vi "Plugin-001-MaterialTest.vi"(0 "Configuration Page":refnum<class "Material-ConfigPage.lvclass">, 11 "error in":errorcluster) -> (15 "error out":errorcluster)   [LabVIEW 2013, in "Material-RunTest.lvclass"]
doc: "DisplayName=\"Deploy Configuration Template\"\nDescription=\"This VI serves as a template page for the Deploy Configuration UI.\""
uses:
  Plugins/Run Material Test/Material-RunTest.lvclass
  Material-ConfigPage.lvclass
  Reuse Library/featherweight/Core/Sequencer/FTW-Sequencer.lvclass/FTW-Sequencer.ctl
  Plugins/Run Material Test/Material-RunTest.lvclass/Material-RunTest.ctl
  <vilib>/Utility/miscctls.llb/LVPointTypeDef.ctl
  Reuse Library/featherweight/Core/Regex/FTW-Regex.vi
  Reuse Library/featherweight/Core/Error/FTW-ERR-StatusException.vi
  Reuse Library/featherweight/Core/Error/FTW-ERR-ThrowError.vi
  Reuse Library/featherweight/Core/Sequencer/FTW-Sequencer.lvclass
  Reuse Library/featherweight/Core/Messaging/Message.Actor/FTW-Message-Actor.lvclass
  <instrlib>/Keyence LK-G5000/Keyence LK-G5000.lvlib
  <instrlib>/Keyence LK-G5000/Public/Constant/Comm Interface.ctl
  Plugins/Motion Control/Motion-ControlAll.lvclass
  Reuse Library/Database API/Database-API.lvclass
panel:
  out "Overall Sheet Passed?":bool
  out "Total Average Thickness of Sheet":dbl format="%_6g"
  out "Average Thickness Line 3":dbl format="%_5g"
  out "Average Thickness Line 2":dbl format="%_5g"
  out "Average Thickness Line 1":dbl format="%_5g"
  out "Thickness Measured Real Time":sgl format="%_6g"
  in  "Begin Test":bool
  out "Line 3 test passed?":bool
  out "Line 2 test passed?":bool
  out "Line 1 test passed?":bool
  out "Mixed Signal Graph":T1(graph)
  out "Message Received":string
  # "Inputs"
  # "Outputs"
  # "First Plugin"
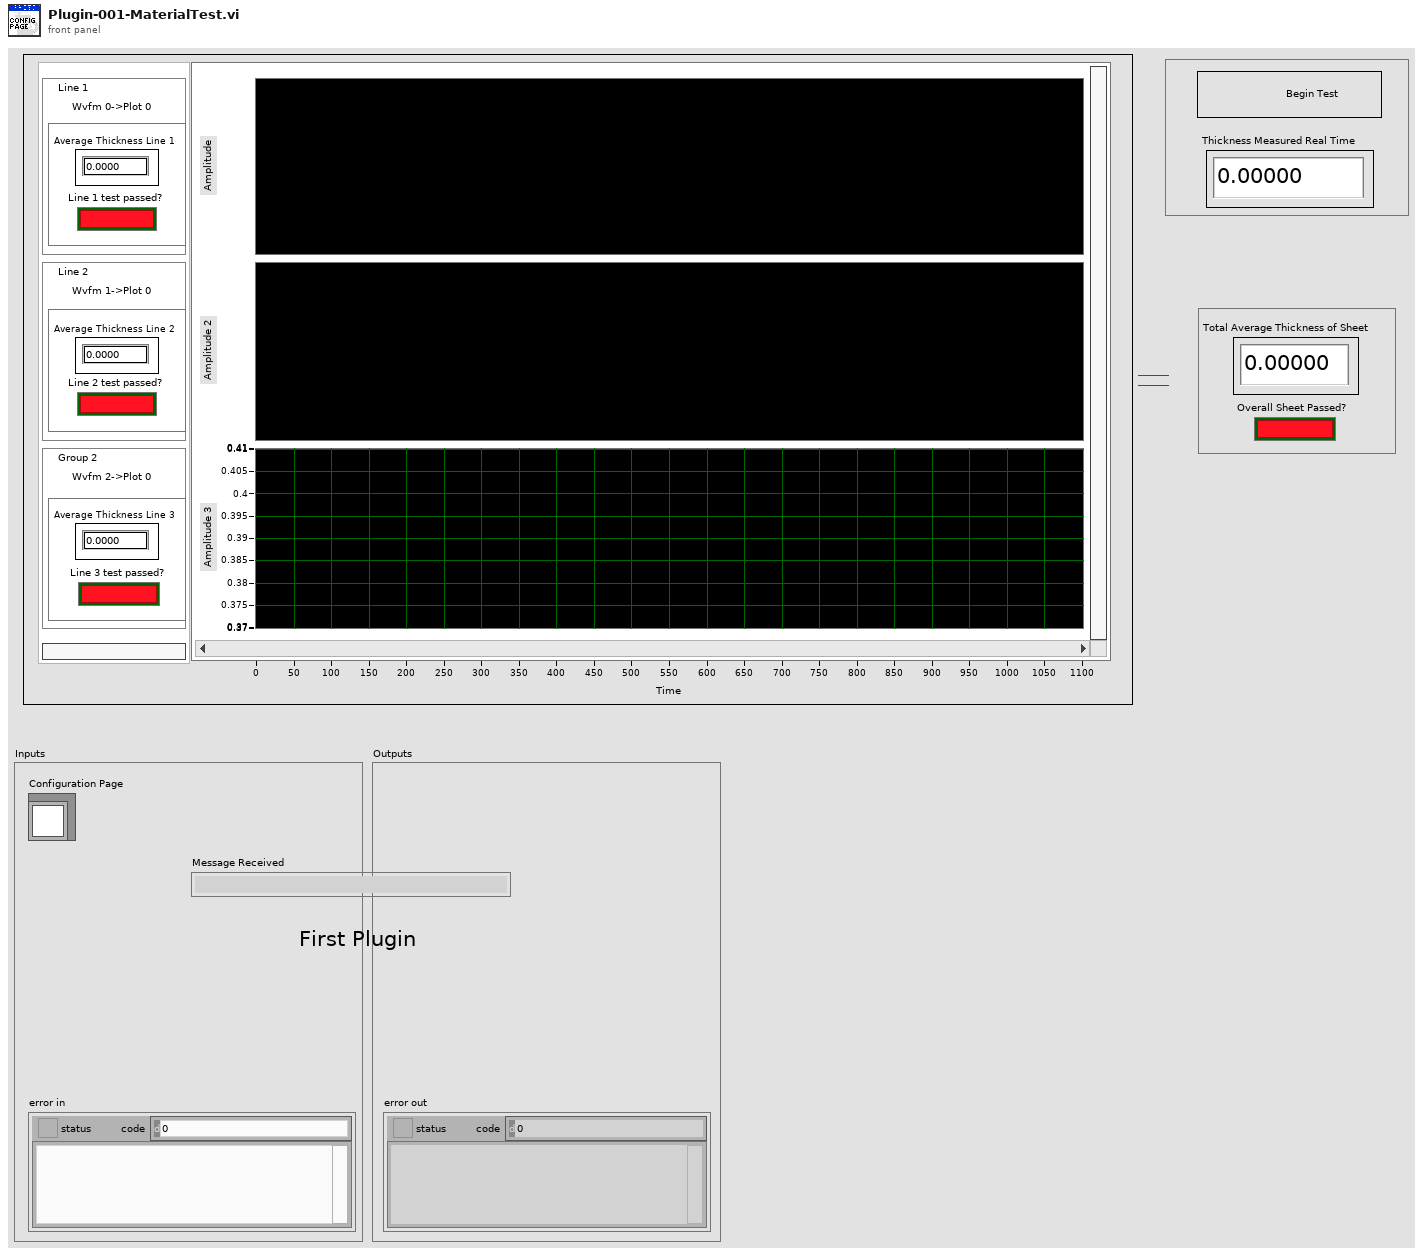
[diagram p1: front panel]
types:
  T1 = cluster{waveform(sgl), waveform(sgl), waveform(sgl)}
  T2 = typedef "Keyence LK-G5000.lvlib/Comm Interface.ctl" = enum8{"USB", "ETHERNET"}
  T3 = typedef "LVPointTypeDef.ctl" = cluster{"Horizontal":i16, "Vertical":i16}
  T4 = cluster{"PageCommands":refnum<event-registration>}
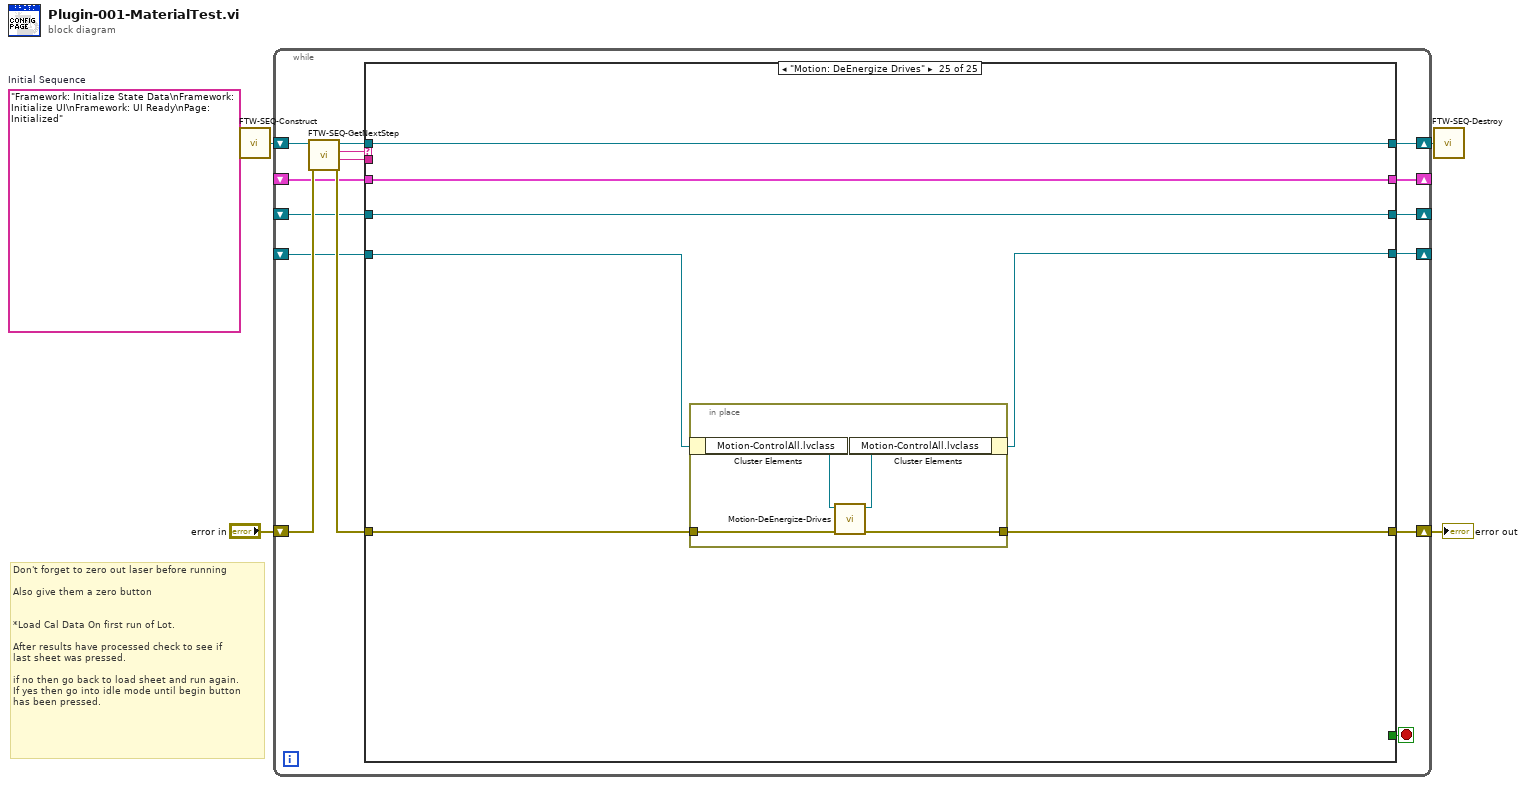
[diagram p0: block diagram]
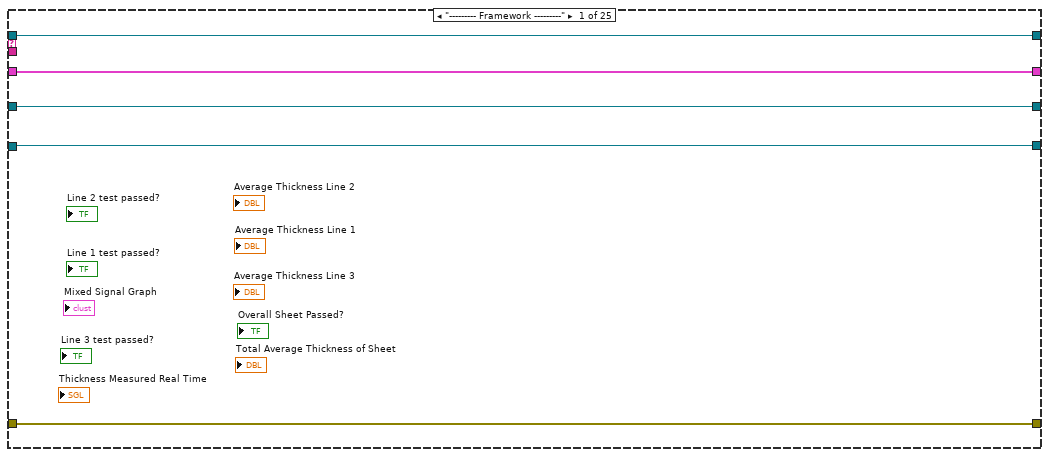
[diagram p2: hidden frame]
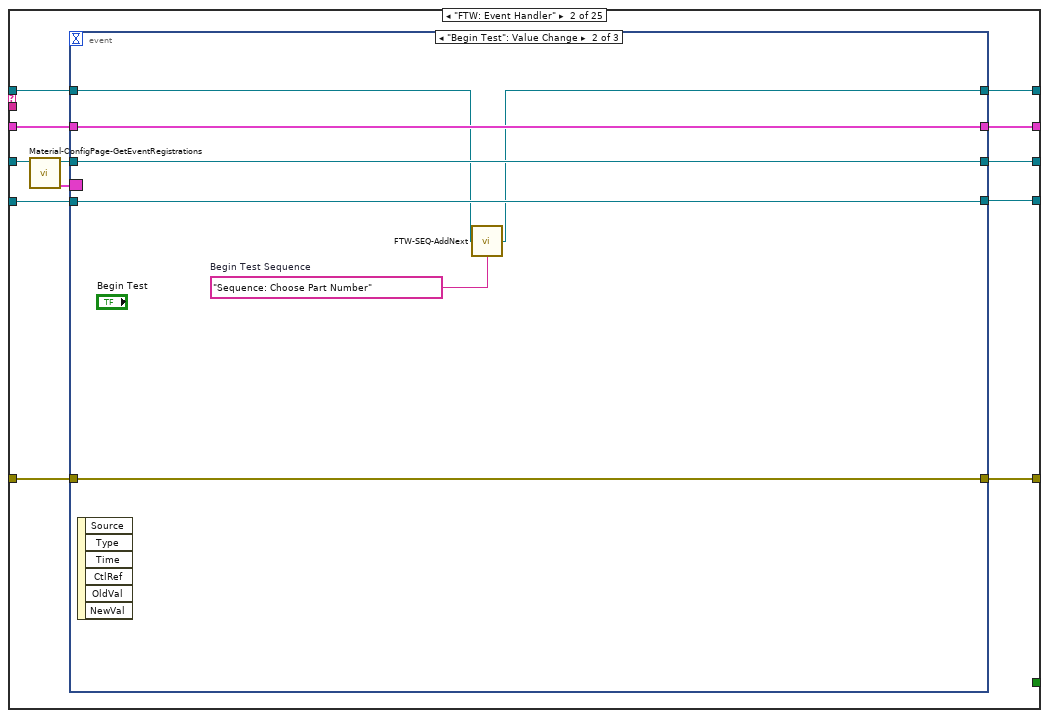
[diagram p3: hidden frame]
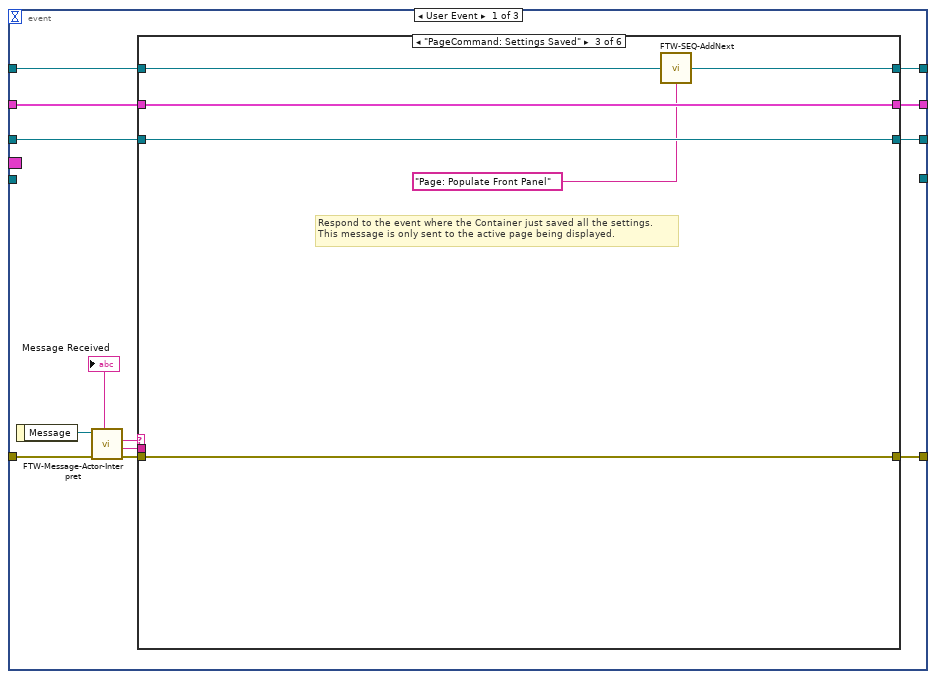
[diagram p4: hidden frame]
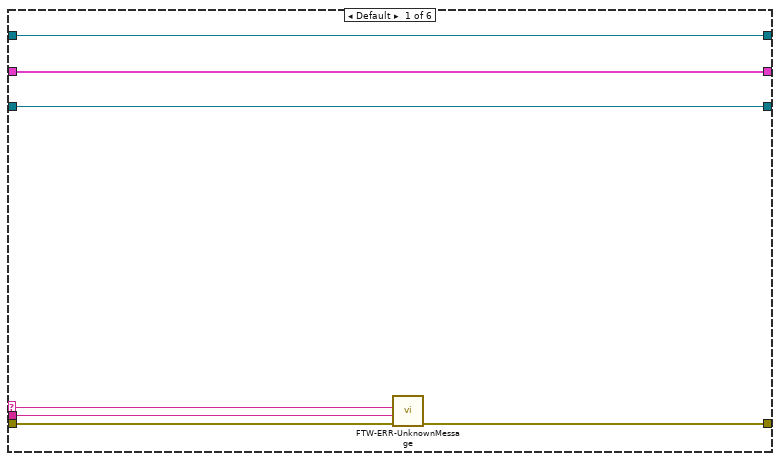
[diagram p5: hidden frame]
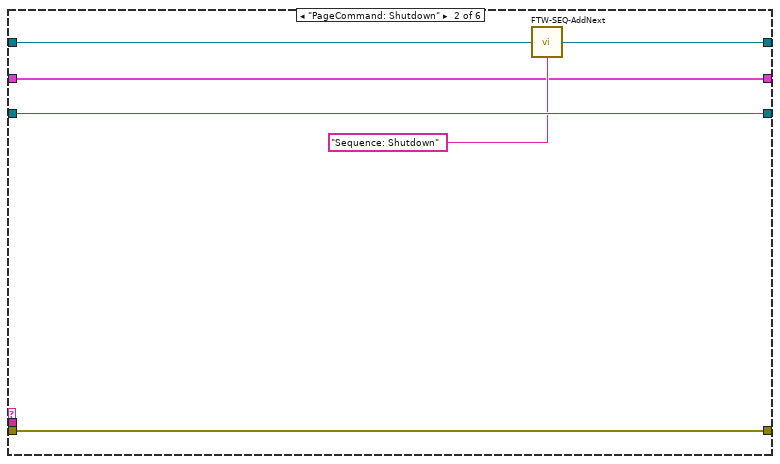
[diagram p6: hidden frame]
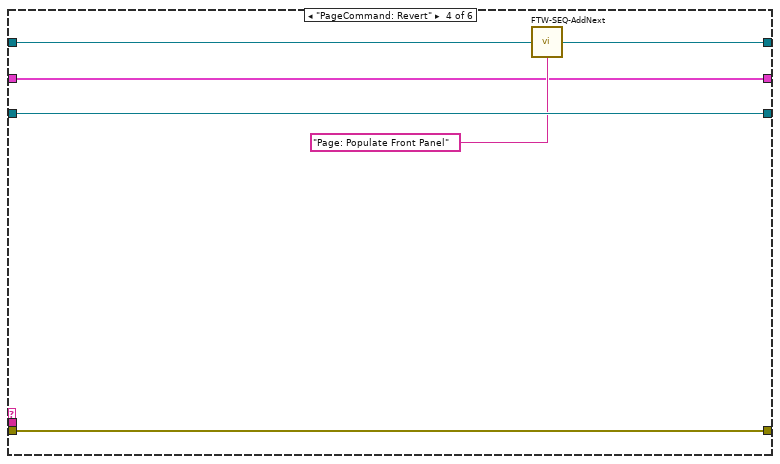
[diagram p7: hidden frame]
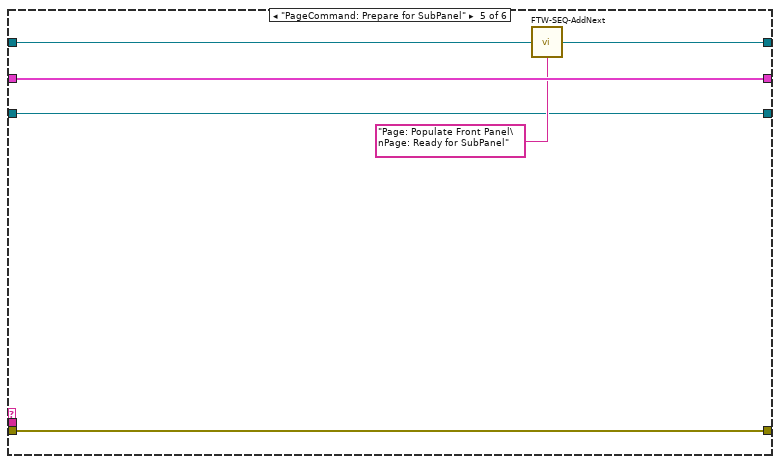
[diagram p8: hidden frame]
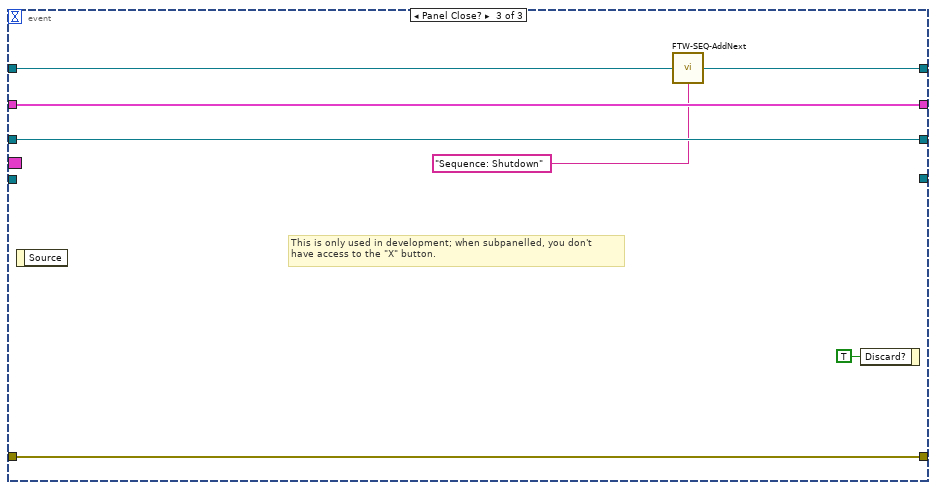
[diagram p10: hidden frame]
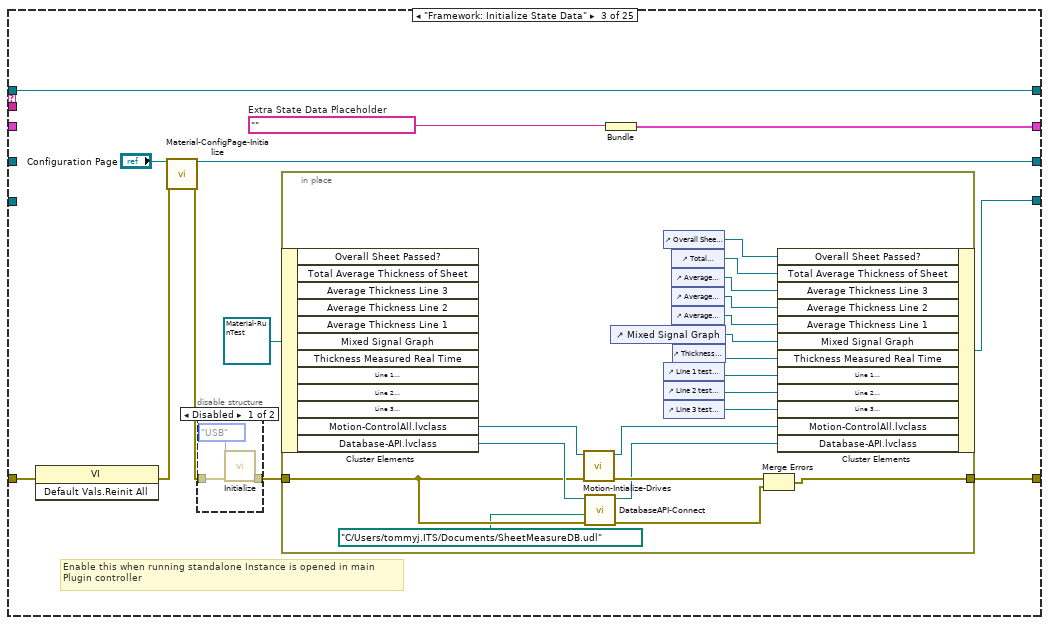
[diagram p11: hidden frame]
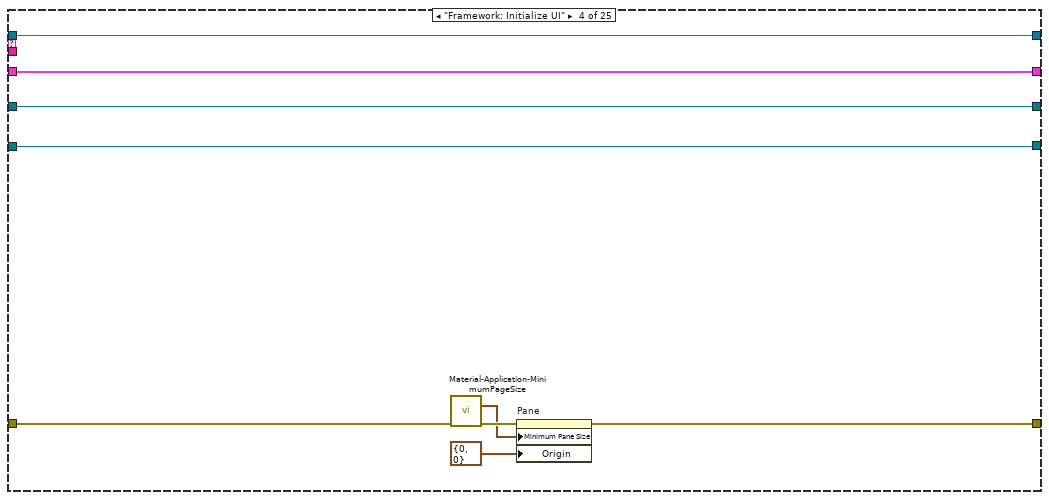
[diagram p13: hidden frame]
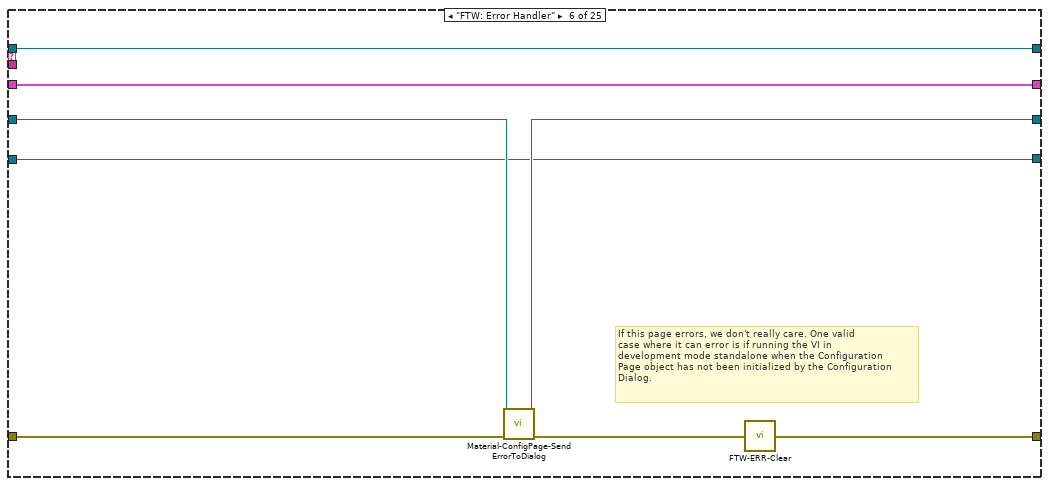
[diagram p15: hidden frame]
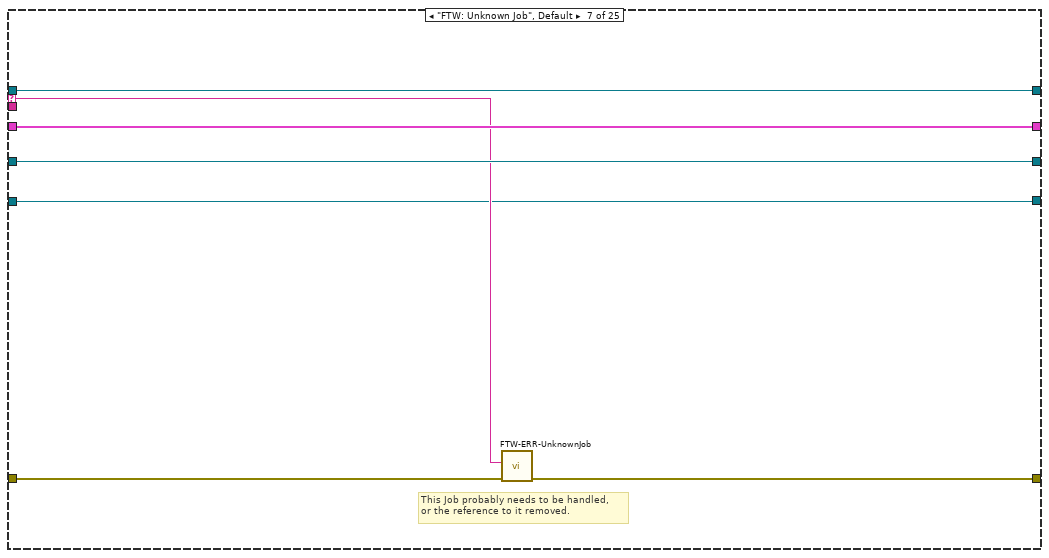
[diagram p16: hidden frame]
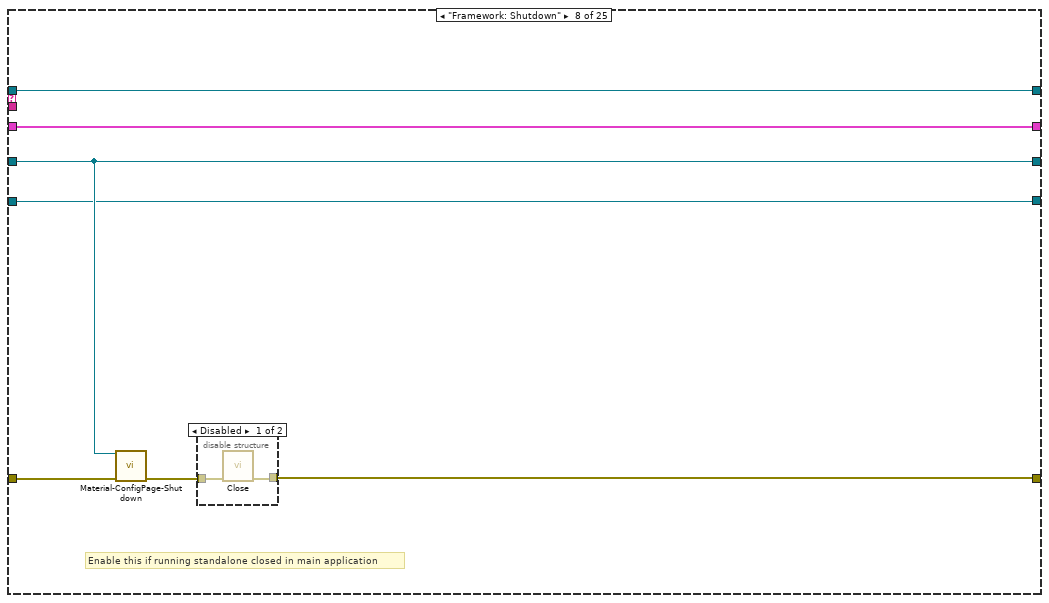
[diagram p17: hidden frame]
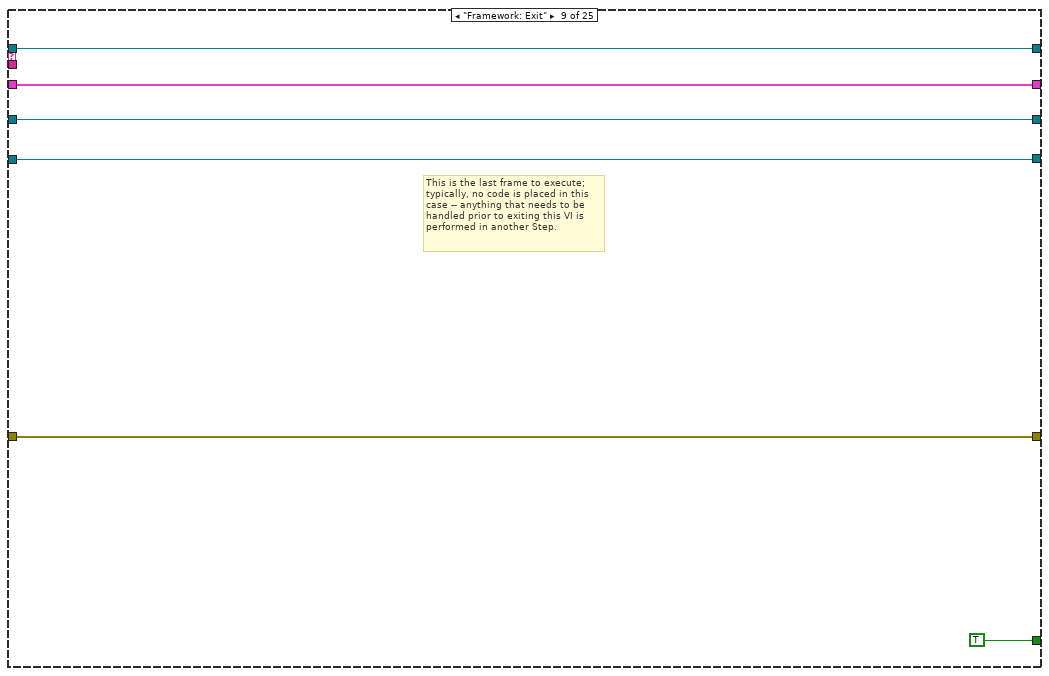
[diagram p19: hidden frame]
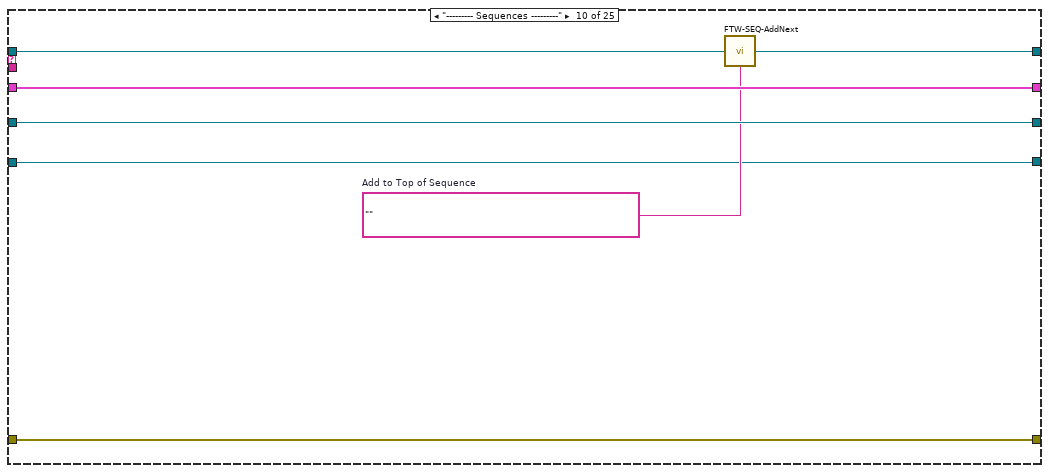
[diagram p20: hidden frame]
diagram:
  w5 = "Framework: Initialize State Data\nFramework: Initialize UI\nFramework: UI Ready\nPage: Initialized"  # Initial Sequence
  # "Don't forget to zero out laser before running\n\nAlso give them a zero button\n\n\n*Load Cal Data On first run of Lot.\n\nAfter results have processed check to see if\nlast sheet was pressed. \n\nif no then go back to load sheet and run again. \nIf yes then go into idle mode until begin button\nhas been pressed."
  n1 = call "FTW-SEQ-Construct.vi"("Initial Sequence"=w5) -> ("Sequencer"=w4:refnum<class "FTW-Sequencer.lvclass">)
  n2 = while {
    shift-right: [w18] -> w3
    shift-left: w4 -> [w9]
    shift-right: [w19] -> w2
    shift-left: "error in" -> [w17]
    shift-right: [w13] -> _
    shift-left: _ -> [w12]
    shift-right: [w11] -> _
    shift-left: _ -> [w10]
    shift-right: [w7] -> _
    shift-left: _ -> [w6]
    stop <- w14 stop-if-true
    n3 = call "FTW-SEQ-GetNextStep.vi"("error in"=w17, "Sequencer"=w9) -> ("error out"=w20:errorcluster, "Job Data"=w8:string, "Current Job"=w15:string, "Sequencer out"=w16:refnum<class "FTW-Sequencer.lvclass">)  [unwired: 6 in]
    n4 = case shown="\"Motion: DeEnergize Drives\"" w15 {
      selector: w15 -> [_ _ _ _ _ _ w157 _ _ _ _ _ _ _ _ _ _ _ _ _ _ _ _ _ _]
      tunnel: [w23 w35 w101 w138 w147 w154 w159 w163 w176 w184 w191 w197 w209 w230 w251 w258 w265 w276 w289 w295 w299 w308 w310 w315 w326] -> w19
      tunnel: w20 -> [w23 w34 w106 w139 w147 w151 w160 w167 w176 w184 w191 w200 w208 w233 w253 w260 w267 w278 w289 w296 w299 w309 w310 w318 w329]
      tunnel: w16 -> [w24 w37 w109 w137 w144 w149 w162 w168 w174 w181 w188 w202 w214 w235 w254 w261 w268 w273 w286 w292 w302 w304 w313 w320 w331]
      tunnel: [w24 w36 w109 w137 w144 w149 w162 w168 w174 w180 w187 w201 w214 w235 w254 w261 w268 w274 w286 w292 w302 w304 w313 w320 w331] -> w18
      tunnel: [_ _ _ _ _ _ _ _ TRUE _ _ _ _ _ _ _ _ _ _ _ _ _ _ _ _] -> w14
      tunnel: [w25 w33 w110 w142 w146 w155 w161 w169 w177 w185 w192 w204 w216 w237 w256 w263 w270 w280 w288 w297 w301 w307 w314 w321 w332] -> w13
      tunnel: w12 -> [w25 w31 _ w142 w146 w155 w161 w169 w177 w185 w192 w204 w216 w237 w256 w263 w270 w280 w288 w297 w301 w307 w314 w321 w332]
      tunnel: [w22 w32 w102 w135 w145 w152 w158 w166 w175 w183 w190 w203 w215 w236 w255 w262 w269 w279 w287 w293 w300 w305 w312 w319 w330] -> w11
      tunnel: w10 -> [w22 w30 _ w135 w145 w153 w158 w166 w175 w183 w190 w203 w215 w236 w255 w262 w269 w279 w287 w294 w300 w306 w312 w319 w330]
      tunnel: w8 -> [_ _ _ _ _ _ _ _ _ _ _ _ _ _ _ _ _ _ _ _ _ _ _ _ _]
      tunnel: [w21 w26 w99 w134 w143 w148 w156 w165 w173 w179 w186 w198 w210 w229 w250 w257 w264 w271 w285 w290 w298 w303 w311 w316 w327] -> w7
      tunnel: w6 -> [w21 w27 _ w134 w143 w148 w156 w165 w173 w179 w186 w199 w213 w234 w252 w259 w266 w277 w285 w290 w298 w303 w311 w317 w328]
      frame "--------- Framework ---------" {
      }
      frame "FTW: Event Handler" {
        n5 = call "Material-ConfigPage-GetEventRegistrations.vi"("Configuration Page"=w30) -> ("Events"=w28:T4, "Configuration Page out"=w29:refnum<class "Material-ConfigPage.lvclass">)  [unwired: 9 in]
        n6 = event shown="[1] \"Begin Test\": Value Change" {
          selector: w28 -> [_ _ _]
          dyn-events: _ -> [_ _ _]
          timeout: _ -> [_ _ _]
          tunnel: w37 -> [w43 w88 w93]
          tunnel: [w44 w87 w92] -> w36
          tunnel: [w48 w85 w96] -> w35
          tunnel: w34 -> [w49 w85 w96]
          tunnel: [w42 w91 w97] -> w33
          tunnel: w31 -> [w41 w91 w97]
          tunnel: w29 -> [w46 w89 w95]
          tunnel: [w45 w89 w95] -> w32
          tunnel: [_ w90 _] -> w26
          tunnel: w27 -> [_ w90 _]
          event User Event {
            n7 = event-data() -> ("Message"=w39:refnum<class "FTW-Message.lvclass">)  [unwired: 1 in]
            n8 = call "FTW-Message-Actor-Interpret.vi"("error in"=w49, "Message"=w39) -> ("error out"=w47:errorcluster, "Sender"=w38:string, "Parameter"=w40:string)  [unwired: 6 in, 1 out]
            "Message Received" <- w40
            n9 = case shown="\"PageCommand: Settings Saved\"" w40 {
              selector: w40 -> [w51 _ _ _ _ _]
              tunnel: [w55 w62 w68 w74 w75 w81] -> w48
              tunnel: w47 -> [w56 w62 w68 w74 w75 w81]
              tunnel: w46 -> [w54 w61 w67 w73 w76 w82]
              tunnel: [w54 w61 w67 w73 w76 w82] -> w45
              tunnel: [w53 w57 w65 w71 w79 w83] -> w44
              tunnel: w43 -> [w53 w60 w66 w72 w80 w83]
              tunnel: [w52 w58 w64 w69 w78 w84] -> w42
              tunnel: w41 -> [w52 w58 w64 w69 w78 w84]
              tunnel: w38 -> [w50 _ _ _ _ _]
              frame Default {
                n10 = call "FTW-ERR-UnknownMessage.vi"("error in"=w56, "Sender"=w50, "Unknown Parameter"=w51) -> ("error out"=w55:errorcluster)  [unwired: 8 in]
              }
              frame "PageCommand: Shutdown" {
                n11 = call "FTW-SEQ-AddNext.vi"("Add Next in Sequence"="Sequence: Shutdown", "Sequencer"=w60) -> ("Sequencer out"=w57:refnum<class "FTW-Sequencer.lvclass">)  [unwired: 2 in]
              }
              frame "PageCommand: Settings Saved" {
                # "Respond to the event where the Container just saved all the settings.\nThis message is only sent to the active page being displayed."
                n12 = call "FTW-SEQ-AddNext.vi"("Add Next in Sequence"="Page: Populate Front Panel" ("Add to Top of Sequence"), "Sequencer"=w66) -> ("Sequencer out"=w65:refnum<class "FTW-Sequencer.lvclass">)  [unwired: 2 in]
              }
              frame "PageCommand: Revert" {
                n13 = call "FTW-SEQ-AddNext.vi"("Add Next in Sequence"="Page: Populate Front Panel", "Sequencer"=w72) -> ("Sequencer out"=w71:refnum<class "FTW-Sequencer.lvclass">)  [unwired: 2 in]
              }
              frame "PageCommand: Prepare for SubPanel" {
                n14 = call "FTW-SEQ-AddNext.vi"("Add Next in Sequence"="Page: Populate Front Panel\nPage: Ready for SubPanel", "Sequencer"=w80) -> ("Sequencer out"=w79:refnum<class "FTW-Sequencer.lvclass">)  [unwired: 2 in]
              }
              frame "PageCommand: Displayed" {
                # "This case is important for dynamically-registering\nVI Server objects for events, since that operation\nwould fail if the Front Panel is not currently being shown.\nThis is because, those references have not yet been constructed."
              }
            }
          }
          event "Begin Test": Value Change {
            w86 = "Sequence: Choose Part Number"  # Begin Test Sequence
            n15 = event-data() -> ()  [unwired: 1 in, 6 out]
            n16 = call "FTW-SEQ-AddNext.vi"("Add Next in Sequence"=w86, "Sequencer"=w88) -> ("Sequencer out"=w87:refnum<class "FTW-Sequencer.lvclass">)  [unwired: 2 in]
          }
          event Panel Close? {
            # "This is only used in development; when subpanelled, you don't\nhave access to the \"X\" button."
            n17 = event-data() -> ()  [unwired: 1 in, 1 out]
            n18 = call "FTW-SEQ-AddNext.vi"("Add Next in Sequence"="Sequence: Shutdown" ("Add to Top of Queue"), "Sequencer"=w93) -> ("Sequencer out"=w92:refnum<class "FTW-Sequencer.lvclass">)  [unwired: 2 in]
            n19 = event-data("Discard?"=TRUE) -> ()  [unwired: 1 in, 1 out]
          }
        }
      }
      frame "Framework: Initialize State Data" {
        w108 = ""  # Extra State Data Placeholder
        # "Enable this when running standalone Instance is opened in main\nPlugin controller"
        n20 = invoke class="VI" method="Default Vals.Reinit All"(error in=w106) -> (error out=w105:errorcluster)  [unwired: 2 in, 2 out]
        n21 = call-dynamic "Material-ConfigPage-Initialize.vi"("Configuration Page"="Configuration Page", "error in"=w105) -> ("Configuration Page out"=w102:refnum<class "Material-ConfigPage.lvclass">, "error out"=w104:errorcluster)  [unwired: 12 in]
        n22 = disable-structure shown="Disabled" {
          disable-tunnel: w104 -> [w112 w114]
          disable-tunnel: [w111 w114] -> w103
          frame Disabled {
            n23 = call <instrlib>:"Initialize.vi"("error in (no error)"=w112, "Comm Interface"=Comm_Interface."USB") -> ("error out"=w111:errorcluster)  [unwired: 9 in]
          }
          frame Enabled {
          }
        }
        n24 = in-place {
          in-place-border: w103 -> [w120]
          in-place-border: [w116] -> w101
          n25 = in-place-cluster #1(refnum<class "Material-RunTest.lvclass"> refnum ("Material-RunTest.lvclass")) -> ("Motion-ControlAll.lvclass"=w133:refnum<class "Motion-ControlAll.lvclass">, "Database-API.lvclass"=w121:refnum<class "Database-API.lvclass">)  [unwired: 10 out]
          n26 = call "Motion-Intialize-Drives.vi"("error in (no error)"=w120, "Motion-ControlAll in"=w133) -> ("error out"=w119:errorcluster, "Motion-ControlAll out"=w132:refnum<class "Motion-ControlAll.lvclass">)  [unwired: 8 in]
          n27 = call "DatabaseAPI-Connect.vi"("error in (no error)"=w120, "Database (mdb)  File Path"=path "C:/Users/tommyj.ITS/Documents/SheetMeasureDB.udl", "Database-API in"=w121) -> ("error out"=w118:errorcluster, "Database-API out"=w117:refnum<class "Database-API.lvclass">)  [unwired: 7 in]
          n28 = control-ref of="Mixed Signal Graph"() -> (w131:refnum<vi>)
          n29 = control-ref of="Overall Sheet Passed?"() -> (w122:refnum<vi>)
          n30 = control-ref of="Line 1 test passed?"() -> (w129:refnum<vi>)
          n31 = control-ref of="Line 2 test passed?"() -> (w128:refnum<vi>)
          n32 = control-ref of="Line 3 test passed?"() -> (w127:refnum<vi>)
          n33 = control-ref of="Total Average Thickness of Sheet"() -> (w123:refnum<vi>)
          n34 = control-ref of="Average Thickness Line 3"() -> (w124:refnum<vi>)
          n35 = control-ref of="Average Thickness Line 2"() -> (w125:refnum<vi>)
          n36 = control-ref of="Average Thickness Line 1"() -> (w126:refnum<vi>)
          n37 = control-ref of="Thickness Measured Real Time"() -> (w130:refnum<vi>)
          n38 = Merge Errors(w119, w118) -> (w116:errorcluster)
          n39 = in-place-cluster #1("Overall Sheet Passed?"=w122, "Total Average Thickness of Sheet"=w123, "Average Thickness Line 3"=w124, "Average Thickness Line 2"=w125, "Average Thickness Line 1"=w126, "Mixed Signal Graph"=w131, "Thickness Measured Real Time"=w130, "Line 1\ntest passed?"=w129, "Line 2\ntest passed?"=w128, "Line 3\ntest passed?"=w127, "Motion-ControlAll.lvclass"=w132, "Database-API.lvclass"=w117) -> (w99:refnum<class "Material-RunTest.lvclass">)
        }
        n40 = Bundle("Extra State Data Placeholder"=w108) -> (w110:cluster{"Extra State Data Placeholder":string})  [unwired: 1 in]
      }
      frame "Framework: Initialize UI" {
        n41 = call "Material-Application-MinimumPageSize.vi"("error in"=w139) -> ("Minimum Pane Size"=w140:cluster{"Horizontal":i16, "Vertical":i16}, "error out"=w141:errorcluster)  [unwired: 13 in]
        n42 = property on="Pane" class="Pane"(error in=w141, "Minimum Pane Size"=w140, "Origin"=T3 {"Horizontal"=0, "Vertical"=0}) -> (error out=w138:errorcluster)  [unwired: 1 in, 1 out]
      }
      frame "Framework: UI Ready" {
      }
      frame "FTW: Error Handler" {
        # "If this page errors, we don't really care. One valid\ncase where it can error is if running the VI in\ndevelopment mode standalone when the Configuration\nPage object has not been initialized by the Configuration\nDialog."
        n43 = call "Material-ConfigPage-SendErrorToDialog.vi"("Configuration Page in"=w153, "error in"=w151) -> ("Configuration Page out"=w152:refnum<class "Material-ConfigPage.lvclass">, "error out"=w150:errorcluster)  [unwired: 12 in]
        n44 = call "FTW-ERR-Clear.vi"("error to snuff"=w150) -> ("no error"=w154:errorcluster)
      }
      frame "FTW: Unknown Job", Default {
        # "This Job probably needs to be handled,\nor the reference to it removed."
        n45 = call "FTW-ERR-UnknownJob.vi"("error in"=w160, "Unknown Job"=w157) -> ("error out"=w159:errorcluster)  [unwired: 9 in]
      }
      frame "Framework: Shutdown" {
        # "Enable this if running standalone closed in main application"
        n46 = call "Material-ConfigPage-Shutdown.vi"("Configuration Page"=w166, "error in"=w167) -> ("error out"=w164:errorcluster)  [unwired: 13 in]
        n47 = disable-structure shown="Disabled" {
          disable-tunnel: w164 -> [w171 w172]
          disable-tunnel: [w170 w172] -> w163
          frame Disabled {
            n48 = call <instrlib>:"Close.vi"("error in (no error)"=w171) -> ("error out"=w170:errorcluster)  [unwired: 10 in]
          }
          frame Enabled {
          }
        }
      }
      frame "Framework: Exit" {
        # "This is the last frame to execute;\ntypically, no code is placed in this\ncase -- anything that needs to be\nhandled prior to exiting this VI is\nperformed in another Step."
      }
      frame "--------- Sequences ---------" {
        w182 = ""  # Add to Top of Sequence
        n49 = call "FTW-SEQ-AddNext.vi"("Add Next in Sequence"=w182, "Sequencer"=w181) -> ("Sequencer out"=w180:refnum<class "FTW-Sequencer.lvclass">)  [unwired: 2 in]
      }
      frame "Sequence: Shutdown" {
        w189 = "Framework: Shutdown\nFramework: Exit"  # Framework Shutdown
        n50 = call "FTW-SEQ-AddNext.vi"("Add Next in Sequence"=w189, "Sequencer"=w188) -> ("Sequencer out"=w187:refnum<class "FTW-Sequencer.lvclass">)  [unwired: 2 in]
      }
      frame "Sequence: Choose Part Number" {
        n51 = call "Material-ChoosePart#-Spec.vi"("error in (no error)"=w200, "Material-RunTest.lvclass"=w199) -> ("error out"=w197:errorcluster, "Cancel Test"=w195:bool, "Invalid Spec Values"=w196:bool, "Material-RunTest.lvclass out"=w198:refnum<class "Material-RunTest.lvclass">)  [unwired: 6 in]
        n52 = Or(x=w196, y=w195) -> (x .or. y?=w193:bool)
        n53 = case shown="False" w193 {
          tunnel: ["Motion: Energize Drives\nSequence: Load Sheet\nSequence: Line 1 Test\nSequence: Line 2 Test\nSequence: Line 3 Test\nSequence: Record Test Results" ("Add Next in Sequence") "" ("Add Next in Sequence")] -> w194
          frame False {
          }
          frame True {
          }
        }
        n54 = call "FTW-SEQ-AddNext.vi"("Add Next in Sequence"=w194, "Sequencer"=w202) -> ("Sequencer out"=w201:refnum<class "FTW-Sequencer.lvclass">)  [unwired: 2 in]
      }
      frame "Sequence: Load Sheet" {
        n55 = invoke class="VI" method="Default Vals.Reinit All"(error in=w208) -> (error out=w207:errorcluster)  [unwired: 2 in, 2 out]
        n56 = in-place {
          in-place-border: w207 -> [w228]
          in-place-border: [w217] -> w212
          n57 = in-place-cluster #2(w213) -> ("Motion-ControlAll.lvclass"=w227:refnum<class "Motion-ControlAll.lvclass">)
          n58 = call "Motion-Move-XandY.vi"("Y Drive Acc/Speed/Velocity"="MA1: A 10: V 20: AD 10: D ", "X Drive Acc/Speed/Velocity"="MA1: A 10: V 20: AD 10: D ", "error in (no error)"=w228, "X Coordinates"="-880000", "Y Coordinates"="880000", "Motion-ControlAll in"=w227) -> ("error out"=w225:errorcluster, "Motion-ControlAll out"=w226:refnum<class "Motion-ControlAll.lvclass">)  [unwired: 4 in]
          n59 = call "Motion-PollAxis-Main.vi"("error in (no error)"=w225, "Motion-ControlAll in"=w226) -> ("error out"=w224:errorcluster, "Motion-ControlAll out"=w223:refnum<class "Motion-ControlAll.lvclass">)  [unwired: 8 in]
          n60 = in-place-cluster #2("Motion-ControlAll.lvclass"=w223) -> (w211:refnum<class "Material-RunTest.lvclass">)
          n61 = call "Material-VacuumControl.vi"("error in (no error)"=w224, "Vacuum On/Off"=TRUE) -> ("error out"=w217:errorcluster)  [unwired: 9 in]
        }
        n62 = call "Material-LoadSheet-Dialog.vi"("error in"=w212, "Material-RunTest.lvclass in"=w211) -> ("error out"=w209:errorcluster, "Material-RunTest.lvclass out"=w210:refnum<class "Material-RunTest.lvclass">)  [unwired: 8 in]
      }
      frame "Sequence: unLoad Sheet" {
        n63 = invoke class="VI" method="Default Vals.Reinit All"(error in=w233) -> (error out=w232:errorcluster)  [unwired: 2 in, 2 out]
        n64 = in-place {
          in-place-border: w232 -> [w249]
          in-place-border: [w238] -> w231
          n65 = in-place-cluster #3(w234) -> ("Motion-ControlAll.lvclass"=w248:refnum<class "Motion-ControlAll.lvclass">)
          n66 = call "Motion-Move-XandY.vi"("Y Drive Acc/Speed/Velocity"="MA1: A 10: V 20: AD 10: D ", "X Drive Acc/Speed/Velocity"="MA1: A 10: V 20: AD 10: D ", "error in (no error)"=w249, "X Coordinates"="-880000", "Y Coordinates"="880000", "Motion-ControlAll in"=w248) -> ("error out"=w246:errorcluster, "Motion-ControlAll out"=w247:refnum<class "Motion-ControlAll.lvclass">)  [unwired: 4 in]
          n67 = call "Motion-PollAxis-Main.vi"("error in (no error)"=w246, "Motion-ControlAll in"=w247) -> ("error out"=w245:errorcluster, "Motion-ControlAll out"=w244:refnum<class "Motion-ControlAll.lvclass">)  [unwired: 8 in]
          n68 = in-place-cluster #3("Motion-ControlAll.lvclass"=w244) -> (w229:refnum<class "Material-RunTest.lvclass">)
          n69 = call "Material-VacuumControl.vi"("error in (no error)"=w245, "Vacuum On/Off"=FALSE) -> ("error out"=w238:errorcluster)  [unwired: 9 in]
        }
        n70 = call "Material-Dialog-UnloadSheet.vi"("error in (no error)"=w231) -> ("error out"=w230:errorcluster)  [unwired: 10 in]
      }
      frame "Sequence: Line 1 Test" {
        n71 = call "Material-Line1-TestMain.vi"("error in (no error)"=w253, "Material-RunTest in"=w252) -> ("error out"=w251:errorcluster, "Material-RunTest out"=w250:refnum<class "Material-RunTest.lvclass">)  [unwired: 8 in]
      }
      frame "Sequence: Line 2 Test" {
        n72 = call "Material-Line2-TestMain.vi"("error in (no error)"=w260, "Material-RunTest in"=w259) -> ("error out"=w258:errorcluster, "Material-RunTest out"=w257:refnum<class "Material-RunTest.lvclass">)  [unwired: 8 in]
      }
      frame "Sequence: Line 3 Test" {
        n73 = call "Material-Line3-TestMain.vi"("error in (no error)"=w267, "Material-RunTest in"=w266) -> ("error out"=w265:errorcluster, "Material-RunTest out"=w264:refnum<class "Material-RunTest.lvclass">)  [unwired: 8 in]
      }
      frame "Sequence: Process Results" {
        n74 = call "Material-ProcessResults.vi"("error in (no error)"=w278, "Material-RunTest in"=w277) -> ("error out"=w276:errorcluster, "Material-RunTest out"=w275:refnum<class "Material-RunTest.lvclass">)  [unwired: 8 in]
        n75 = in-place {
          in-place-border: [w282] -> w272
          n76 = in-place-cluster #4(w275) -> ("Last Sheet in Lot"=w281:bool)
          n77 = case shown="True" w281 {
            tunnel: ["Sequence: unLoad Sheet\nMotion: Energize Drives\nSequence: Load Sheet\nSequence: Line 1 Test\nSequence: Line 2 Test\nSequence: Line 3 Test\nSequence: Record Test Results" ("Add Next in Sequence") "Sequence: unLoad Sheet\nMotion: DeEnergize Drives" ("Add Next in Sequence")] -> w282
            frame False {
            }
            frame True {
              # "Unload the sheet: the test\nis finished for specified lot"
            }
          }
          n78 = in-place-cluster #4("Last Sheet in Lot"=w281) -> (w271:refnum<class "Material-RunTest.lvclass">)
        }
        n79 = call "FTW-SEQ-AddNext.vi"("Add Next in Sequence"=w272, "Sequencer"=w273) -> ("Sequencer out"=w274:refnum<class "FTW-Sequencer.lvclass">)  [unwired: 2 in]
      }
      frame "--------- Application Logic ---------" {
      }
      frame "Page: Initialized" {
        w291 = TRUE  # Allow user to open Diagram from SubPanel?
        n80 = call "Material-ConfigPage-Initialized.vi"("Configuration Page"=w294, "Allow user to open Diagram from SubPanel?"=w291, "error in"=w296) -> ("Configuration Page out"=w293:refnum<class "Material-ConfigPage.lvclass">, "error out"=w295:errorcluster)  [unwired: 11 in]
      }
      frame "Page: Populate Front Panel" {
      }
      frame "Page: Ready for SubPanel" {
        n81 = call "Material-ConfigPage-ReadyForSubPanel.vi"("Configuration Page"=w306, "error in"=w309) -> ("Configuration Page out"=w305:refnum<class "Material-ConfigPage.lvclass">, "error out"=w308:errorcluster)  [unwired: 12 in]
      }
      frame "--------- Motion Control ---------" {
      }
      frame "Motion: Energize Drives" {
        n82 = in-place {
          in-place-border: w318 -> [w325]
          in-place-border: [w322] -> w315
          n83 = in-place-cluster #5(w317) -> ("Motion-ControlAll.lvclass"=w324:refnum<class "Motion-ControlAll.lvclass">)
          n84 = call "Motion-Energize-Drives.vi"("error in (no error)"=w325, "Motion-ControlAll in"=w324) -> ("error out"=w322:errorcluster, "Motion-ControlAll out"=w323:refnum<class "Motion-ControlAll.lvclass">)  [unwired: 8 in]
          n85 = in-place-cluster #5("Motion-ControlAll.lvclass"=w323) -> (w316:refnum<class "Material-RunTest.lvclass">)
        }
      }
      frame "Motion: DeEnergize Drives" {
        n86 = in-place {
          in-place-border: w329 -> [w336]
          in-place-border: [w333] -> w326
          n87 = in-place-cluster #6(w328) -> ("Motion-ControlAll.lvclass"=w335:refnum<class "Motion-ControlAll.lvclass">)
          n88 = call "Motion-DeEnergize-Drives.vi"("error in (no error)"=w336, "Motion-ControlAll in"=w335) -> ("error out"=w333:errorcluster, "Motion-ControlAll out"=w334:refnum<class "Motion-ControlAll.lvclass">)  [unwired: 8 in]
          n89 = in-place-cluster #6("Motion-ControlAll.lvclass"=w334) -> (w327:refnum<class "Material-RunTest.lvclass">)
        }
      }
    }
  }
  "error out" <- w2
  n90 = call "FTW-SEQ-Destroy.vi"("Sequencer"=w3) -> ()  [unwired: 1 in]
